vi "LocalSearcher Qname.vi"() -> (3 "QName":string)   [LabVIEW 2013]
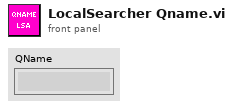
[diagram p1: front panel]
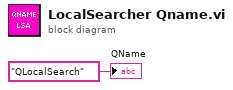
[diagram p0: block diagram]
diagram:
  "QName" <- "QLocalSearch" ("name (unnamed)")
